vi "Actor Core.vi"(8 "error in":errorcluster caption="错误输入", 11 "硬件 in":refnum<class "硬件.lvclass"> caption="操作者输入") -> (0 "error out":errorcluster caption="错误输出", 3 "Actor out":refnum<class "Actor.lvclass"> caption="操作者输出")   [LabVIEW 2015, in "硬件.lvlib" / "硬件.lvclass"]
doc: "(<B>文件名</B>: Actor Framework.lvlib:Actor.lvclass:Actor Core.vi)\n\n接收发送至操作者的消息，响应消息并处理可能导致操作者关闭的错误。\n\n子孙类重写该VI，使操作者完成特定的任务。使用调用父方法节点实现重写。"
uses:
  <vilib>/ActorFramework/Actor/Actor.lvclass
panel:
  out "已发送":string
  out "接收到的":string
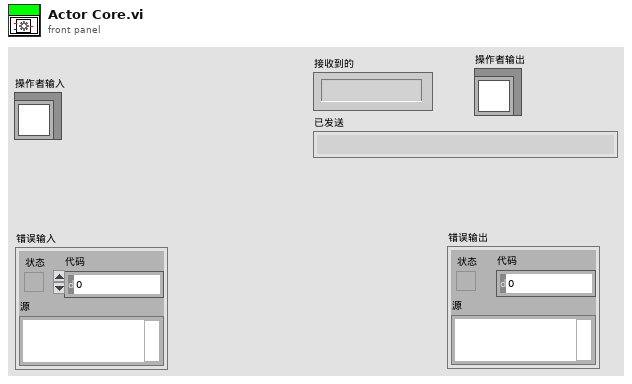
[diagram p1: front panel]
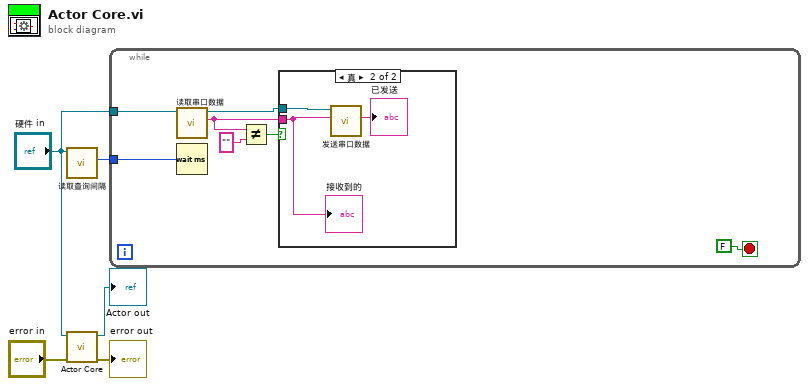
[diagram p0: block diagram]
diagram:
  n1 = call-dynamic "读取查询间隔.vi"("硬件输入"="硬件 in") -> ("查询间隔"=w1:u32)  [unwired: 8 in, 2 out]
  n2 = call-parent "Actor Core.vi"("error in"="error in", "Actor in"="硬件 in") -> ("error out"=→"error out":errorcluster, "Actor out"=→"Actor out":refnum<class "Actor.lvclass">)  [unwired: 8 in]
  n3 = while {
    tunnel: "硬件 in" -> [w11]
    tunnel: w1 -> [w6]
    stop <- FALSE stop-if-true
    n4 = call-dynamic "读取串口数据.vi"("硬件 输入"=w11) -> ("读取到的内容"=w7:string, "硬件 输出"=w9:refnum<class "硬件.lvclass">)  [unwired: 8 in, 1 out]
    n5 = Wait (ms)(milliseconds to wait=w6) -> ()  [unwired: 1 out]
    n6 = Not Equal?(x=w7, y="") -> (x != y?=w8:bool)
    n7 = case shown="真" w8 {
      tunnel: w9 -> [_ w15]
      tunnel: w7 -> [_ w14]
      frame False {
      }
      frame True {
        n8 = call-dynamic "发送串口数据.vi"("原始数据"=w14, "硬件 输入"=w15) -> ("已发送"=→"已发送":string)  [unwired: 7 in, 2 out]
        "接收到的" <- w14
      }
    }
  }
